vi "clFileReader_getLenght.vi"(11 "clFileReader.lvclass IN":refnum<class "clFileReader.lvclass">) -> (0 "blocklen":u32, 3 "clFileReader.lvclassOut":refnum<class "clFileReader.lvclass">)   [LabVIEW 2016, in "vi_lib.lvlib" / "clFileReader.lvclass"]
uses:
  clFileReader.lvclass
  clFileReader.lvclass/clFileReader.ctl
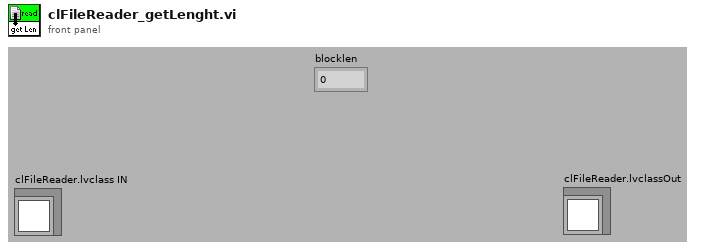
[diagram p1: front panel]
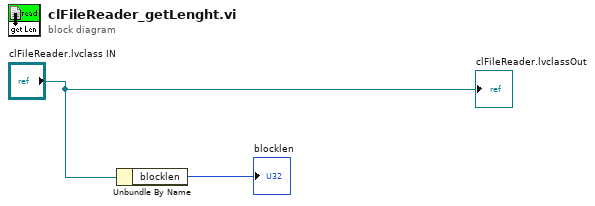
[diagram p0: block diagram]
diagram:
  n1 = Unbundle By Name("clFileReader.lvclass IN") -> ("blocklen"=→"blocklen":u32)
  "clFileReader.lvclassOut" <- "clFileReader.lvclass IN"
